vi "action.vi"(0 "HGF_SVVarManVisitor_create in":refnum<class "HGF_SVVarManVisitor_create.lvclass">, 2 "HGF_Visitable":refnum<class "HGF_Visitable.lvclass">, 5 "error in (no error)":errorcluster) -> (14 "HGF_SVVarManVisitor_create out":refnum<class "HGF_SVVarManVisitor_create.lvclass">, 16 "dup HGF_Visitable":refnum<class "HGF_Visitable.lvclass">, 19 "error out":errorcluster)   [LabVIEW 2012, in "HGF_SV.lvlib" / "HGF_SVVarManVisitor_create.lvclass"]
doc: "This is a dynamic dispatch VI that is called from Visitor.visit(). It will call member VIs of Visitable to perform the requested action which means: calling public methods of Visitable child class.\n\n<B>Hint:</B> This method is abstract and need to be implemented by child classes."
uses:
  HGF_SVVarManVisitor_create.lvclass
  HGF_BaseClasses/HGF_Visitable/HGF_Visitable.lvclass
  HGF_DSC/HGF_DSCVarManager/HGF_DSCVarManager.lvclass
  HGF_BaseClasses/HGF_Visitor/HGF_Visitor.lvclass
  HGF_SVVarManVisitor_create.lvclass/HGF_SVVarManVisitor_create.ctl
  HGF_BaseClasses/HGF_TriggeredEvent/HGF_TriggeredEvent.lvclass
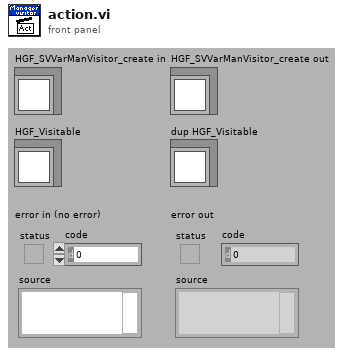
[diagram p1: front panel]
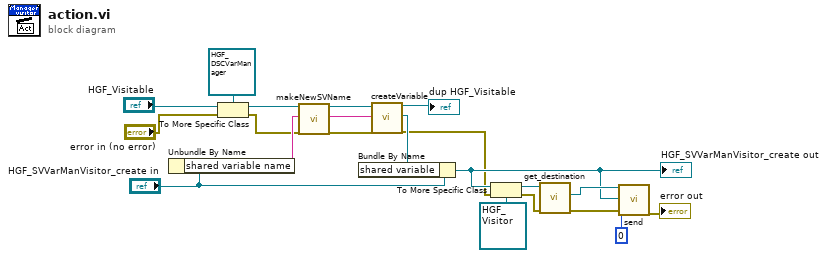
[diagram p0: block diagram]
diagram:
  n1 = Unbundle By Name("HGF_SVVarManVisitor_create in") -> ("shared variable name"=w15:string)
  n2 = To More Specific Class(target class=refnum<class "HGF_DSCVarManager.lvclass"> refnum ("DSC.lvlib:HGF_DSCVarManager.lvclass"), reference="HGF_Visitable", error in="error in (no error)") -> (specific class reference=w20:refnum<class "HGF_DSCVarManager.lvclass">, error out=w11:errorcluster)
  n3 = call "makeNewSVName.vi"("HGF_DSCVarManager in"=w20, "SV"=w15, "error in (no error)"=w11) -> ("HGF_DSCVarManager out"=w19:refnum<class "HGF_DSCVarManager.lvclass">, "SV out"=w13:string, "error out"=w12:errorcluster)  [unwired: 14 in]
  n4 = call-dynamic "createVariable.vi"("HGF_DSCVarManager in"=w19, "shared variable name"=w13, "error in (no error)"=w12) -> ("HGF_DSCVarManager out"=→"dup HGF_Visitable":refnum<class "HGF_DSCVarManager.lvclass">, "shared variable"=w14:refnum<k21>, "error out"=w5:errorcluster)  [unwired: 14 in]
  n5 = Bundle By Name(cluster="HGF_SVVarManVisitor_create in", "shared variable"=w14) -> (w6:refnum<class "HGF_SVVarManVisitor_create.lvclass">)
  "HGF_SVVarManVisitor_create out" <- w6
  n6 = To More Specific Class(target class=refnum<class "HGF_Visitor.lvclass"> refnum ("HGF_BaseClasses.lvlib:HGF_Visitor.lvclass"), reference=w6, error in=w5) -> (specific class reference=w8:refnum<class "HGF_Visitor.lvclass">, error out=w4:errorcluster)
  n7 = call "get_destination.vi"("error in (no error)"=w4, "HGF_Visitor"=w8) -> ("error out"=w3:errorcluster, "destination"=w7:refnum<class "HGF_TriggeredEvent.lvclass">)  [unwired: 7 in, 1 out]
  n8 = call-dynamic "send.vi"("HGF_Event"=w7, "Object"=w6, "timeout in ms (-1)"=0, "error in (no error)"=w3) -> ("error out"=→"error out":errorcluster)  [unwired: 13 in, 2 out]
